vi "ROI entry-Full plane UI handler.vi"(11 "Whole plane mode ON":bool) -> (0 "error out":errorcluster)   [LabVIEW 2017]
uses:
  ROI Entry screen/Typedefs/ROI input mode.ctl
  ROI Entry screen/Globals/gl_ROI Entry UI globals.vi
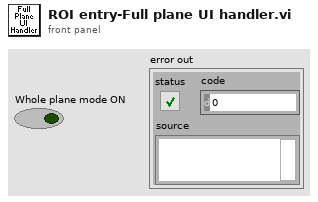
[diagram p1: front panel]
types:
  T1 = enum8{"Enabled", "Disabled", "Disabled and Grayed Out"}
  T2 = typedef "ROI input mode.ctl" = enum16{"Unspecified", "Point-Line-Plane", "Volume"}
  T3 = typedef "ROI entry screen ctrl refs cluster.ctl" = cluster{"Done button":refnum<vi>, "Imaging button":refnum<vi>, "Acquisition button":refnum<vi>, "POI dwell time (us)":refnum<vi>, "Scan dwell time per pixel (us)":refnum<vi>, "# of planes":refnum<vi>, "Zoom Ctrl":refnum<vi>, "Equal size":refnum<vi>, "Channel":refnum<vi>, "Image Display":refnum<vi>, "Z-Plane Selector":refnum<vi>, "Number of lines left":refnum<vi>, "Z-stack folder path":refnum<vi>, "POI Density":refnum<vi>, "Arb Plane Entry":refnum<vi>, "Whole plane":refnum<vi>, "Clear Last":refnum<vi>, "Clear All":refnum<vi>, "Trial Length (sec)":refnum<vi>, "Palette Type":refnum<vi>, "Intensity slider":refnum<vi>, "# POI":refnum<vi>, "Max Z Proj":refnum<vi>, "Zplane ind":refnum<vi>, "Wavelength (nm)":refnum<vi>, "Number of Trials":refnum<vi>, "Funct stim.trig.enable":refnum<vi>, "Funct stim.trig.delay (s)":refnum<vi>, "Line Mode":refnum<vi>, "Step size (µm)":refnum<vi>, "ROI move mode":refnum<vi>, "Cool-down time (s)":refnum<vi>, "Enable cool-down time":refnum<vi>, "Motor Z ind. (um)":refnum<vi>, "AOL Z ind. (um)":refnum<vi>, "Load Reference Image":refnum<vi>}
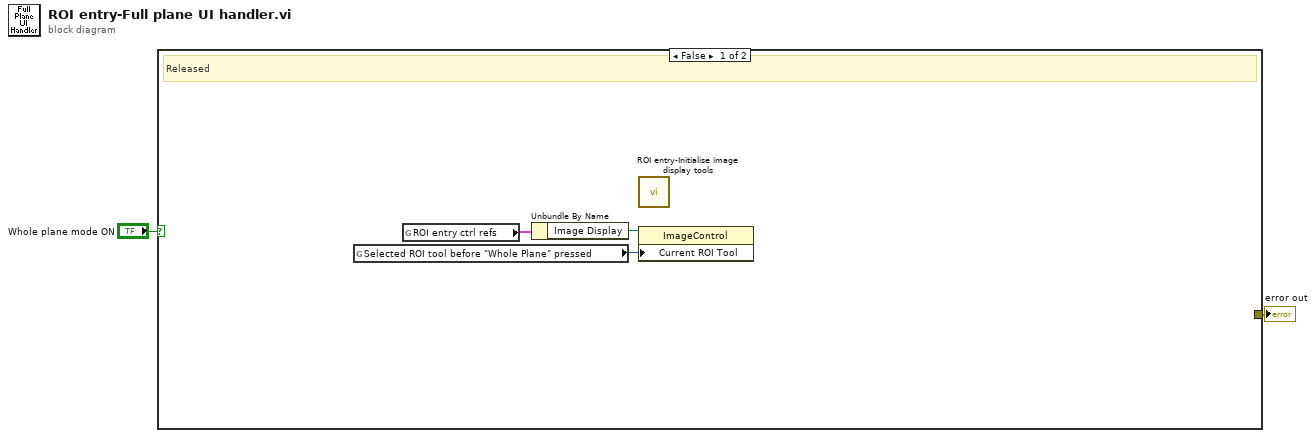
[diagram p0: block diagram]
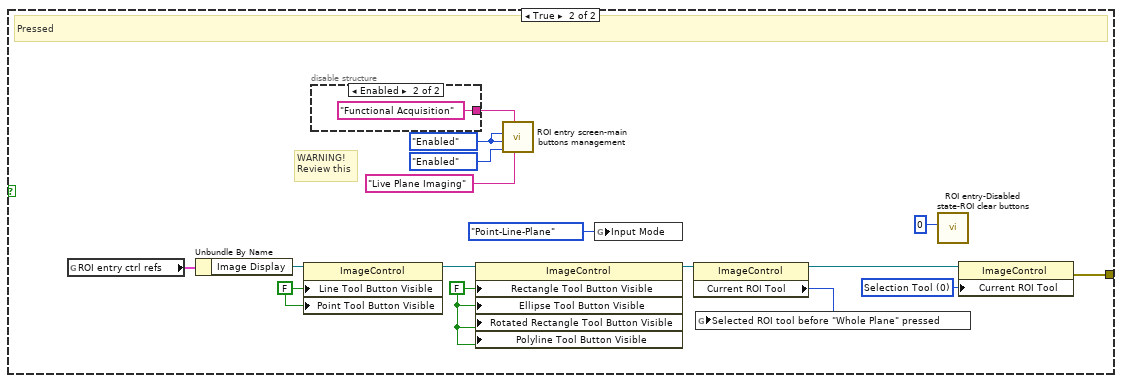
[diagram p2: hidden frame]
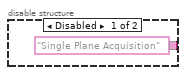
[diagram p3: hidden frame]
diagram:
  n1 = case shown="False" "Whole plane mode ON" {
    tunnel: [_ w9] -> w1
    frame False {
      # "Released"
      n2 = global read "gl_ROI Entry UI globals.vi" "Selected ROI tool before \"Whole Plane\" pressed"() -> (w3:u32)
      n3 = global read "gl_ROI Entry UI globals.vi" "ROI entry ctrl refs"() -> (w5:T3)
      n4 = Unbundle By Name(w5) -> ("Image Display"=w4:refnum<vi>)
      n5 = call "ROI entry-Initialise image display tools.vi"() -> ()  [unwired: 11 in, 1 out]
      n6 = property class="ImageControl"(reference=w4, "Current ROI Tool"=w3) -> ()  [unwired: 1 in, 2 out]
    }
    frame True {
      w19 = u32 0 items=["Zoom Tool"=8, "Selection Tool"=0, "Pan Tool"=9, "Point Tool"=1, "Line Tool"=2, "Rectangle Tool"=3, "Rotated Rectangle Tool"=12, "Polyline Tool"=10, "Polygon Tool"=5, "Freehand Tool"=11, "Closed Freehand Tool"=6, "Ellipse Tool"=4, "Annulus Tool"=7] ("Current ROI Tool")
      w18 = FALSE ("ROI Tool Buttons Visible:Line Tool Button Visible")
      w14 = FALSE ("ROI Tool Buttons Visible:Line Tool Button Visible")
      w13 = T1."Enabled" ("Disabled")
      # "WARNING!\nReview this"
      # "Pressed"
      n7 = global read "gl_ROI Entry UI globals.vi" "ROI entry ctrl refs"() -> (w21:T3)
      n8 = Unbundle By Name(w21) -> ("Image Display"=w20:refnum<vi>)
      n9 = property class="ImageControl"(reference=w20, "Line Tool Button Visible"=w14, "Point Tool Button Visible"=w14) -> (reference out=w15:refnum<vi>)  [unwired: 1 in, 1 out]
      n10 = disable-structure shown="Enabled" {
        disable-tunnel: ["Single Plane Acquisition" ("Boolean Text.Text") "Functional Acquisition" ("Boolean Text.Text")] -> w16
        frame Disabled {
        }
        frame Enabled {
        }
      }
      n11 = property class="ImageControl"(reference=w15, "Rectangle Tool Button Visible"=w18, "Ellipse Tool Button Visible"=w18, "Rotated Rectangle Tool Button Visible"=w18, "Polyline Tool Button Visible"=w18) -> (reference out=w8:refnum<vi>)  [unwired: 1 in, 1 out]
      n12 = call "ROI entry screen-main buttons management.vi"("Imaging button boolean text"="Live Plane Imaging" ("Boolean Text.Text"), "Acquisition button boolean text"=w16, "Imaging button disabled?"=T1."Enabled" ("Disabled"), "Acquisition button disabled?"=w13, "Done button disabled?"=w13) -> ()  [unwired: 7 in]
      n13 = global write "gl_ROI Entry UI globals.vi" "Input Mode"(ROI_input_mode."Point-Line-Plane" ("t")) -> ()
      n14 = property class="ImageControl"(reference=w8) -> (reference out=w7:refnum<vi>, "Current ROI Tool"=w6:u32)  [unwired: 1 in, 1 out]
      n15 = global write "gl_ROI Entry UI globals.vi" "Selected ROI tool before \"Whole Plane\" pressed"(w6) -> ()
      n16 = call "ROI entry-Disabled state-ROI clear buttons.vi"("State"=0) -> ()  [unwired: 10 in, 1 out]
      n17 = property class="ImageControl"(reference=w7, "Current ROI Tool"=w19) -> (error out=w9:errorcluster)  [unwired: 1 in, 1 out]
    }
  }
  "error out" <- w1
